vi "setAllAttributes.vi"(8 "error in (no error)":errorcluster, 10 "attributes":T1(array[cluster]), 11 "xmlNode in":refnum<class "xmlNode.lvclass">) -> (0 "error out":errorcluster, 3 "xmlNode out":refnum<class "xmlNode.lvclass">)   [LabVIEW 2009, in "Tools.lvlib" / "xml.lvlib" / "xmlNode.lvclass"]
doc: "Sets all the xml node Attributes\n\n<xml node attribute1 = \"attribute 1 value\", attribute2 = \"attribute 2 value\">\n <child xml element 1> value </child xml element 1>\n <child xml element 2> value </child xml element 2>\n</xml node>"
uses:
  xmlNode.lvclass
  xmlNode.lvclass/xmlNode.ctl
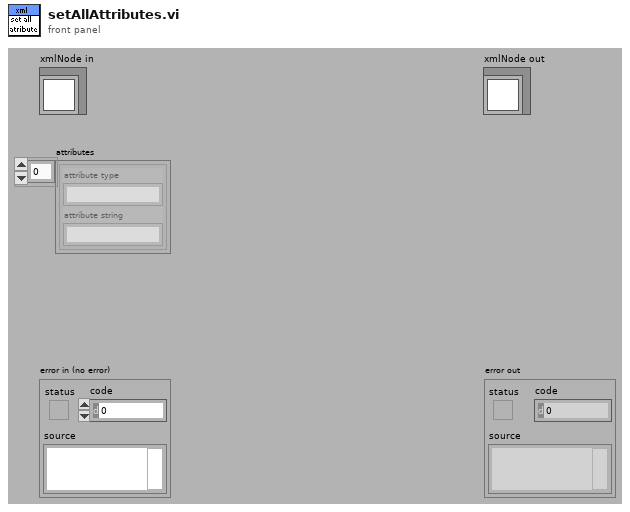
[diagram p1: front panel]
types:
  T1 = cluster{"attribute type":string, "attribute string":string}[]
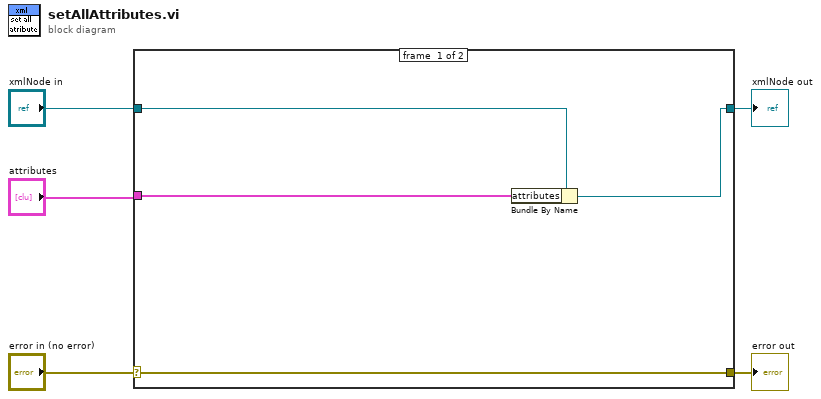
[diagram p0: block diagram]
diagram:
  n1 = case shown="No Error" "error in (no error)" {
    selector: "error in (no error)" -> [w9 w11]
    tunnel: [w9 w11] -> w4
    tunnel: [w6 w10] -> w2
    tunnel: "xmlNode in" -> [w8 w10]
    tunnel: "attributes" -> [w7 _]
    frame #0 {
      n2 = Bundle By Name(cluster=w8, "attributes"=w7) -> (w6:refnum<class "xmlNode.lvclass">)
    }
    frame #1 {
    }
  }
  "error out" <- w4
  "xmlNode out" <- w2
